vi "CMin w AWG.vi"(0 "Semiconductor Module Context":T2, 2 "Measurement Id":string="CMin", 5 "error in (no error)":errorcluster, 6 "VNAs Measurement Parameters":T1) -> (14 "Semiconductor Module Context Out":T2, 19 "error out":errorcluster)   [LabVIEW 2013]
uses:
  <vilib>/NI_TestStand_SemiconductorModule/NI_TestStand_Semiconductor_Module.lvlibp/PinMap/General/SemiconductorModuleContext.ctl
  VNA/VNAs Measurement Parameters.ctl
  <vilib>/NI_TestStand_SemiconductorModule/NI_TestStand_Semiconductor_Module.lvlibp
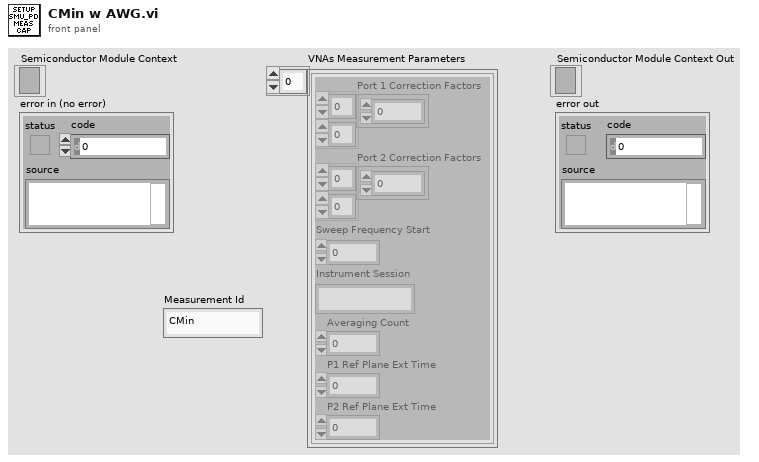
[diagram p1: front panel]
types:
  T1 = typedef "VNAs Measurement Parameters.ctl" = cluster{"Port 1 Correction Factors":cdb[][], "Port 2 Correction Factors":cdb[][], "Sweep Frequency Start":dbl, "Instrument Session":string, "Averaging Count":i32, "P1 Ref Plane Ext Time":dbl, "P2 Ref Plane Ext Time":dbl}[]
  T2 = typedef "NI_TestStand_Semiconductor_Module.lvlibp/SemiconductorModuleContext.ctl" = refnum<k7>
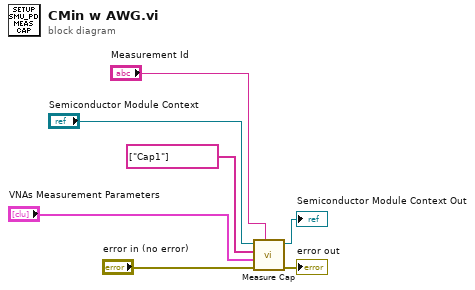
[diagram p0: block diagram]
diagram:
  n1 = call "Measure Cap.vi"("Measurement Id"="Measurement Id", "error in (no error)"="error in (no error)", "VNAs Measurement Parameters"="VNAs Measurement Parameters", "Pins"=string[] ["Cap1"] ("Capacitance Pins"), "Semiconductor Module Context"="Semiconductor Module Context") -> ("error out"=→"error out":errorcluster, "Semiconductor Module Context Out"=→"Semiconductor Module Context Out":T2)  [unwired: 4 in, 1 out]
